vi "Configure Histogram.vi"(0 "VISA resource name":refnum<visa-resource-name>, 1 "Histogram Orientation (0: Horizontal)":i32(ring) items=["Horizontal", "Vertical"], 2 "Histogram Top (5)":dbl=5.0, 3 "Histogram Left (100E-9)":dbl=1e-07, 5 "Histogram Source (1: Channel 1)":i32(ring)=1 items=["Channel 1"=1, "Channel 2"=2, "Channel 3"=3, "Channel 4"=4, "Function 1"=5, "Function 2"=6, "Function 3"=7, "Function 4"=8, "Memory 1"=9, "Memory 2"=10, "Memory 3"=11, "Memory 4"=12, "Differential 1"=61, "Differential 2"=62, "Common 1"=71, "Common 2"=72, "Clock"=15, "MTrend"=16, "MSpectrum"=17, "Equalized"=18], 7 "Histogram Mode (0: Off)":i32(ring) items=["Off", "Waveforms", "Measurement"], 9 "Histogram Size (4.0)":dbl=4.0, 11 "error in (no error)":errorcluster, 12 "Histogram Right (900E-9)":dbl=9e-07, 13 "Histogram Bottom (-1)":dbl=-1.0) -> (4 "VISA resource name out":refnum<visa-resource-name>, 15 "error out":errorcluster)   [LabVIEW 2013, in "Agilent 90000 Series.lvlib"]
doc: "Configures the histogram properties of an oscilloscope. You can configure the histogram type, histogram size and so on."
uses:
  Agilent 90000 Series.lvlib
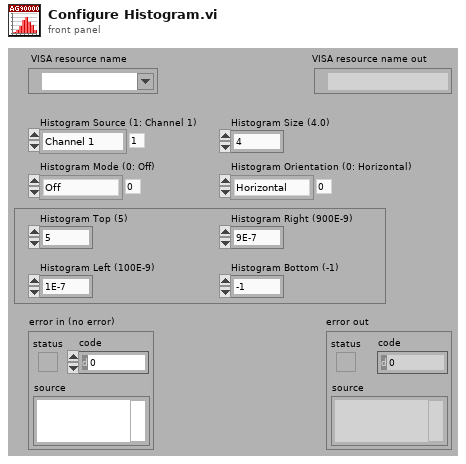
[diagram p1: front panel]
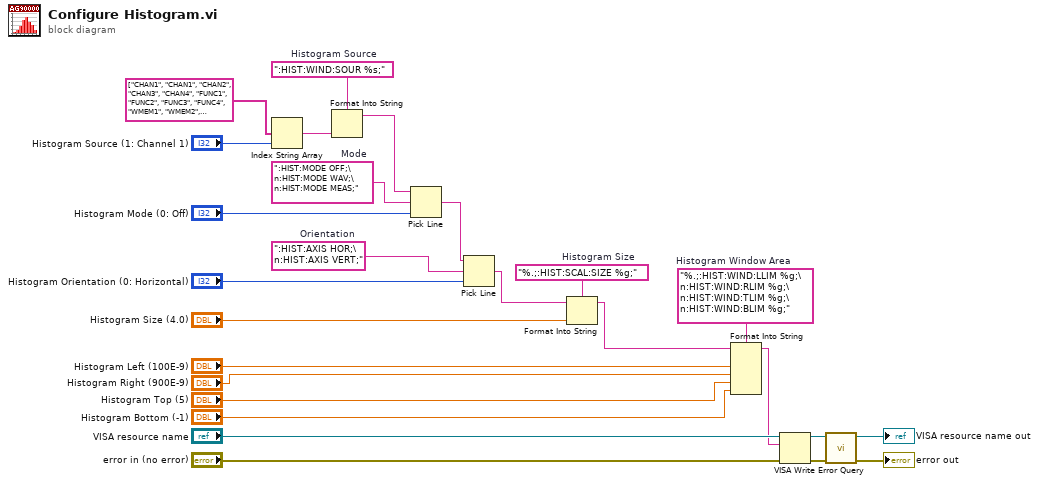
[diagram p0: block diagram]
diagram:
  w7 = "%.;:HIST:WIND:LLIM %g;\n:HIST:WIND:RLIM %g;\n:HIST:WIND:TLIM %g;\n:HIST:WIND:BLIM %g;"  # Histogram Window Area
  w11 = "%.;:HIST:SCAL:SIZE %g;"  # Histogram Size
  w13 = ":HIST:AXIS HOR;\n:HIST:AXIS VERT;"  # Orientation
  w16 = ":HIST:MODE OFF;\n:HIST:MODE WAV;\n:HIST:MODE MEAS;"  # Mode
  w18 = ":HIST:WIND:SOUR %s;"  # Histogram Source
  n1 = Index String Array(1:"Histogram Source (1: Channel 1)", 2:string[] ["CHAN1", "CHAN1", "CHAN2", "CHAN3", "CHAN4", "FUNC1", "FUNC2", "FUNC3", "FUNC4", "WMEM1", "WMEM2", "WMEM3", "WMEM4", "AUX", "LINE", "CLOC", "MTR", "MSP", "EQU", "NONE", "DIG0", "DIG1", "DIG2", "DIG3", "DIG4", "DIG5", "DIG6", "DIG7", "DIG8", "DIG9", "DIG10", "DIG11", "DIG12", "DIG13", "DIG14", "DIG15", "", "", "", "", "", "POD1", "POD2", "", "", "", "", "", "", "", "", "BUS1", "BUS2", "BUS3", "BUS4", "", "", "", "", "", "", "DIFF1", "DIFF2", "", "", "", "", "", "", "", "", "COMM3", "COMM4"]) -> (0:w19:string)  [unwired: 1 out]
  n2 = Format Into String(format string=w18, w19) -> (resulting string=w15:string)  [unwired: 2 in, 1 out]
  n3 = Pick Line(string ("")=w15, multi-line string=w16, line index="Histogram Mode (0: Off)") -> (output string=w12:string)
  n4 = Pick Line(string ("")=w12, multi-line string=w13, line index="Histogram Orientation (0: Horizontal)") -> (output string=w9:string)
  n5 = Format Into String(format string=w11, initial string=w9, "Histogram Size (4.0)") -> (resulting string=w6:string)  [unwired: 1 in, 1 out]
  n6 = Format Into String(format string=w7, initial string=w6, "Histogram Left (100E-9)", "Histogram Right (900E-9)", "Histogram Top (5)", "Histogram Bottom (-1)") -> (resulting string=w2:string)  [unwired: 1 in, 1 out]
  n7 = VISA Write(VISA resource name="VISA resource name", write buffer=w2, error in (no error)="error in (no error)") -> (VISA resource name out=w22:refnum<visa-resource-name>, error out=w21:errorcluster)  [unwired: 1 out]
  n8 = call "Error Query.vi"("error in (no error)"=w21, "VISA resource name"=w22) -> ("error out"=→"error out":errorcluster, "VISA resource name out"=→"VISA resource name out":refnum<visa-resource-name>)  [unwired: 8 out]
